vi "日期字符串格式至时间格式转换(子VI).vi"(11 "data[0]":string) -> (3 "time stamp":timestamp format="%<%Y/%m/%d %H:%M:%S>T")   [LabVIEW 2016, in "数据传输系统.lvlib"]
uses:
  <vilib>/Utility/miscctls.llb/LVDateTimeRec.ctl
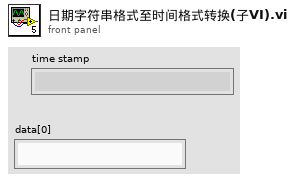
[diagram p1: front panel]
types:
  T1 = typedef "LVDateTimeRec.ctl" = cluster{"fractional second":dbl, "second":i32, "minute":i32, "hour":i32, "day of month":i32, "month":i32, "year":i32, "day of week":i32, "day of year":i32, "DST":i32}
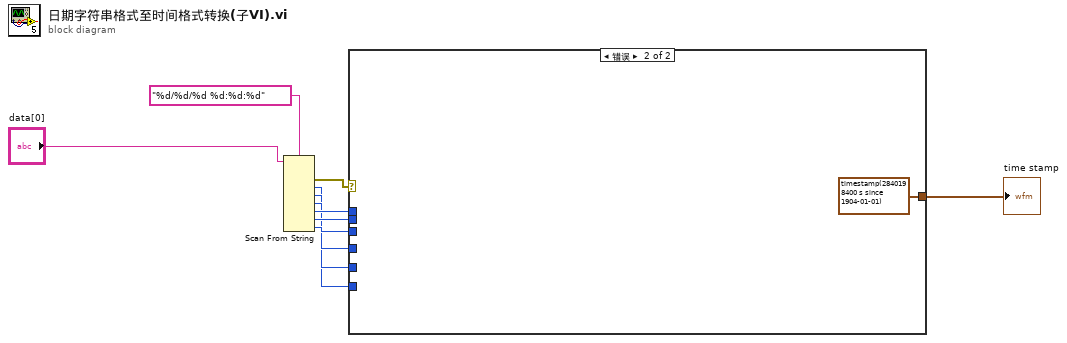
[diagram p0: block diagram]
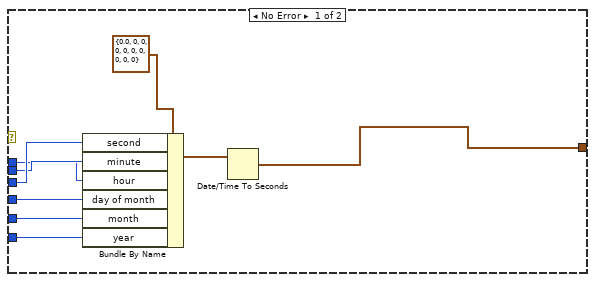
[diagram p2: hidden frame]
diagram:
  n1 = Scan From String(format string="%d/%d/%d %d:%d:%d" ("格式字符串"), input string="data[0]") -> (error out=w2:errorcluster, output 1=w5:i32, output 2=w6:i32, output 3=w7:i32, output 4=w8:i32, output 5=w9:i32, output 6=w10:i32)  [unwired: 8 in, 2 out]
  n2 = case shown="错误" w2 {
    tunnel: w10 -> [w18 _]
    tunnel: w9 -> [w17 _]
    tunnel: w8 -> [w16 _]
    tunnel: w7 -> [w15 _]
    tunnel: w6 -> [w14 _]
    tunnel: w5 -> [w13 _]
    tunnel: [w11 timestamp(2840198400 s since 1904-01-01) ("time stamp")] -> w1
    frame No Error {
      n3 = Bundle By Name(cluster=T1 {"fractional second"=0.0, "second"=0, "minute"=0, "hour"=0, "day of month"=0, "month"=0, "year"=0, "day of week"=0, "day of year"=0, "DST"=0} ("日期时间记录"), "second"=w18, "minute"=w17, "hour"=w16, "day of month"=w15, "month"=w14, "year"=w13) -> (w19:T1)
      n4 = Date/Time To Seconds(2:w19) -> (0:w11:timestamp)  [unwired: 1 in]
    }
    frame Error {
    }
  }
  "time stamp" <- w1
